vi "Shift Array (SubVI).vi"(9 "shift Y":i32, 10 "shift X+":i32, 11 "Array in":dbl[][](array[numeric])) -> (3 "Array out":dbl[][](array[numeric]))   [LabVIEW 2014]
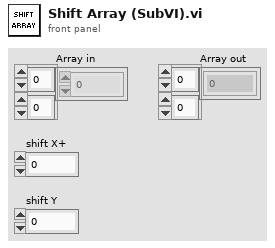
[diagram p1: front panel]
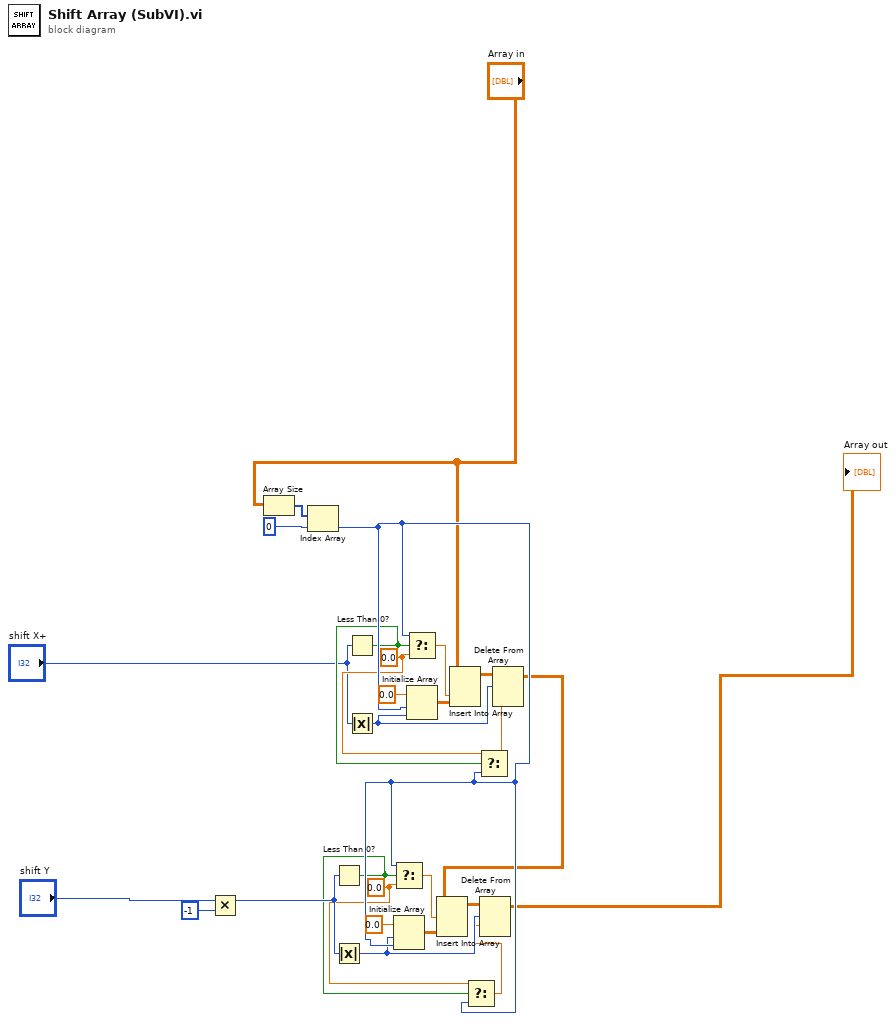
[diagram p0: block diagram]
diagram:
  w18 = 0.0 ("f")
  w12 = 0.0 ("f")
  n1 = Multiply(x="shift Y", y=-1) -> (x*y=w25:i32)
  n2 = Array Size(array="Array in") -> (size(s)=w2:i32[])
  n3 = Index Array(array=w2, index=0) -> (element=w24:i32)
  n4 = Less Than 0?(x=w25) -> (x < 0?=w17:bool)
  n5 = Absolute Value(x=w25) -> (abs(x)=w23:i32)
  n6 = Less Than 0?(x="shift X+") -> (x < 0?=w10:bool)
  n7 = Absolute Value(x="shift X+") -> (abs(x)=w9:i32)
  n8 = Select(t=w24, s=w17, f=w18) -> (s? t:f=w19:dbl)
  n9 = Initialize Array(0.0 ("element"), w23, w24) -> (w14:dbl[][])
  n10 = Select(t=w24, s=w10, f=w12) -> (s? t:f=w8:dbl)
  n11 = Initialize Array(0.0 ("element"), w24, w9) -> (w5:dbl[][])
  n12 = Insert Into Array(array="Array in", index (col)=w8, new element=w5) -> (w6:dbl[][])  [unwired: 1 in]
  n13 = Select(t=w18, s=w17, f=w24) -> (s? t:f=w22:dbl)
  n14 = Select(t=w12, s=w10, f=w24) -> (s? t:f=w11:dbl)
  n15 = Delete From Array(array=w6, length=w9, index (col)=w11) -> (array with subset deleted=w20:dbl[][])  [unwired: 1 in, 1 out]
  n16 = Insert Into Array(array=w20, index (row)=w19, new element=w14) -> (w15:dbl[][])  [unwired: 1 in]
  n17 = Delete From Array(array=w15, length=w23, index (row)=w22) -> (array with subset deleted=→"Array out":dbl[][])  [unwired: 1 in, 1 out]
